vi "Make path absolute.vi"(10 "relative or absolute path":string, 11 "PrintToSingleFileHtml in":refnum<class "PrintToSingleFileHtml.lvclass">) -> (2 "absolute path":path, 3 "PrintToSingleFileHtml out":refnum<class "PrintToSingleFileHtml.lvclass">)   [LabVIEW 2026, in "PrintToSingleFileHtml.lvclass"]
uses:
  PrintToSingleFileHtml.lvclass
  PrintToSingleFileHtml.lvclass/PrintToSingleFileHtml.ctl
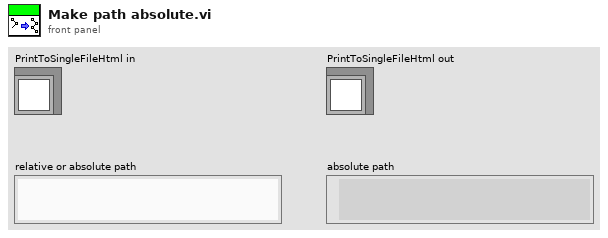
[diagram p1: front panel]
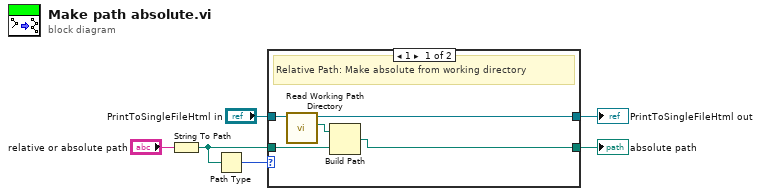
[diagram p0: block diagram]
diagram:
  n1 = String To Path(string="relative or absolute path") -> (path=w2:path)
  n2 = Path Type(1:w2) -> (0:w3:i16)
  n3 = case shown="1" w3 {
    tunnel: w2 -> [w11 w13]
    tunnel: [w10 w13] -> w6
    tunnel: "PrintToSingleFileHtml in" -> [w9 w12]
    tunnel: [w7 w12] -> w1
    frame 1 {
      # "Relative Path: Make absolute from working directory"
      n4 = call-dynamic "Read Working Path Directory.vi"("CoreOperation in"=w9) -> ("Working Path Directory"=w8:path, "CoreOperation out"=w7:refnum<class "PrintToSingleFileHtml.lvclass">)  [unwired: 8 in, 1 out]
      n5 = Build Path(base path=w8, name or relative path=w11) -> (appended path=w10:path)
    }
    frame Default {
      # "Absolute path (or <Not A Path>)"
    }
  }
  "absolute path" <- w6
  "PrintToSingleFileHtml out" <- w1
